vi "Client Main.vi"   [LabVIEW 2020, in "Chat Client.lvclass"]
uses:
  Chat Client.lvclass
panel:
  # "1. Run this VI\n2. Select a user name with the prompt dialog\n3. A chat UI will be launched to send messages to other connected clients.\n4. Once a chat UI is launched this VI can be run again to create a new chat client."
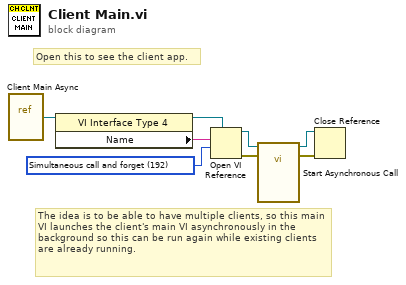
[diagram p0: block diagram]
diagram:
  w3 = 192 items=["Record modifications"=1, "Open templates for editing"=2, "Prompt user to save"=4, "Prepare for reentrant run"=8, "Prompt to find missing subVIs"=16, "Hide loading dialog box"=32, "Enable simultaneous calls"=64, "Prepare to call and forget"=128, "Simultaneous call and forget"=192, "Prepare to call and collect"=256, "Simultaneous call and collect"=320]
  # "Open this to see the client app."
  # "The idea is to be able to have multiple clients, so this main VI launches the client's main VI asynchronously in the background so this can be run again while existing clients are already running."
  n1 = vi-ref "Client Main Async.vi"() -> (w1:refnum<vi>)
  n2 = property class="VI Interface Type 4"(reference=w1) -> (reference out=w4:refnum<vi>, "Name"=w2:string)  [unwired: 1 in, 1 out]
  n3 = Open VI Reference(type specifier VI Refnum (for type only)=w4, vi path=w2, options=w3) -> (vi reference=w6:refnum<vi>, error out=w5:errorcluster)  [unwired: 3 in]
  n4 = call-by-ref "Start Asynchronous Call"(reference=w6, error in=w5) -> (reference out=w8:refnum<vi>, error out=w7:errorcluster)  [unwired: 12 in]
  n5 = Close Reference(reference=w8, error in (no error)=w7) -> ()  [unwired: 1 out]
